vi "Init.vi"(8 "error in (no error)":errorcluster, 11 "Data":variant) -> (0 "error out":errorcluster)   [LabVIEW 2018, in "Outputs.lvlib"]
doc: "This subVI enqueues the named action in to the communications queue along with the input data."
uses:
  Outputs.lvlib
  Private Controls/Module Data.ctl
  Private Controls/Module Action.ctl
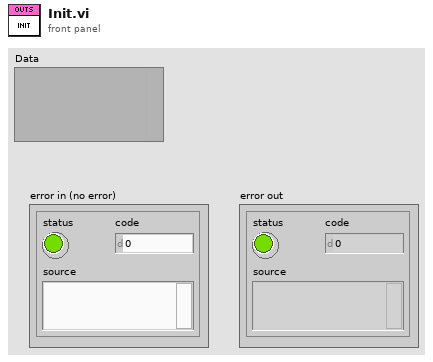
[diagram p1: front panel]
types:
  T1 = typedef "Outputs.lvlib/Module Data.ctl" = cluster{"Data":variant, "Action":T2}
  T2 = typedef "Outputs.lvlib/Module Action.ctl" = enum16{"Init", "Error", "Write 02-06-9265 Vals (AO)", "Write 02-01-9485 Vals (DO)", "Set APU&ECU Cntrls", "Set Bleed-Fuel-ECS Cntrls", "Set ECS Demnd Cluster", "Set Fuel Pres Regltr", "Write Single 02-00-9485 Chann", "Write Single 02-01-9485 Chann"}
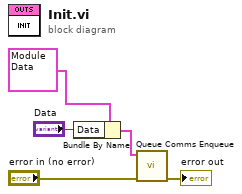
[diagram p0: block diagram]
diagram:
  n1 = Bundle By Name(cluster=T1 {"Data"=variant, "Action"=enum."Init"} ("element"), "Data"="Data") -> (w5:T1)
  n2 = call "Queue Comms Enqueue.vi"("error in (no error)"="error in (no error)", "element"=w5) -> ("error out"=→"error out":errorcluster)  [unwired: 9 in]
